vi "SampleMethod.vi"(8 "error in (no error)":errorcluster, 11 "SampleClass in":refnum<class "SampleClass.lvclass">) -> (0 "error out":errorcluster, 3 "SampleClass out":refnum<class "SampleClass.lvclass">)   [LabVIEW 2020, in "SampleLib.lvlib" / "SampleClass.lvclass"]
uses:
  SampleClass.lvclass
  obj/tests/SampleDependentLib.lvlibp/SampleDependentClass/SampleDependentClass.lvclass
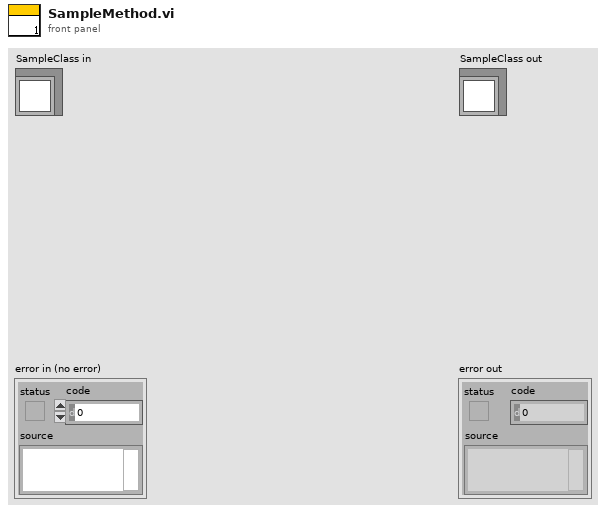
[diagram p1: front panel]
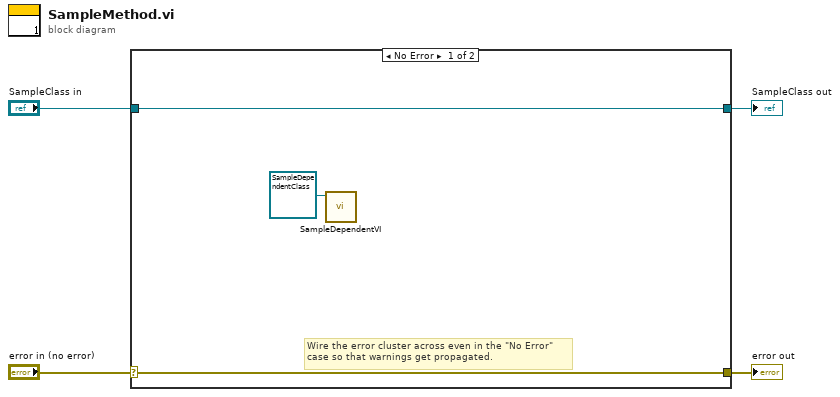
[diagram p0: block diagram]
diagram:
  n1 = case shown="No Error" "error in (no error)" {
    selector: "error in (no error)" -> [w6 w9]
    tunnel: [w6 w9] -> w3
    tunnel: [w7 w8] -> w1
    tunnel: "SampleClass in" -> [w7 w8]
    frame No Error {
      # "Wire the error cluster across even in the \"No Error\"\ncase so that warnings get propagated."
      n2 = call-dynamic "SampleDependentVI.vi"("SampleDependentClass in"=refnum<class "SampleDependentClass.lvclass"> refnum) -> ()  [unwired: 9 in, 2 out]
    }
    frame Error {
    }
  }
  "error out" <- w3
  "SampleClass out" <- w1
